vi "Write Sync Group.vi"(8 "error in (no error)":errorcluster, 10 "Sync Group":u8=128 format="%x", 11 "DriveMotorsLeft in":refnum<class "DriveMotorsLeft.lvclass">) -> (0 "error out":errorcluster, 3 "DriveMotorsLeft out":refnum<class "DriveMotorsLeft.lvclass">)   [LabVIEW 2013, in "DriveMotorsLeft.lvclass"]
uses:
  DriveMotorsLeft.lvclass
  DriveMotorsLeft.lvclass/DriveMotorsLeft.ctl
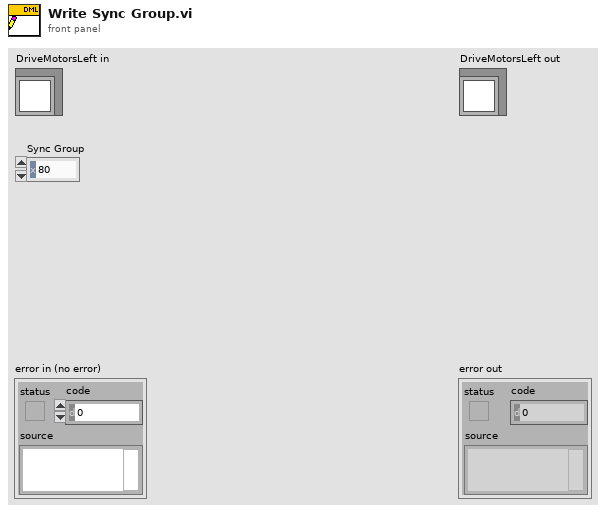
[diagram p1: front panel]
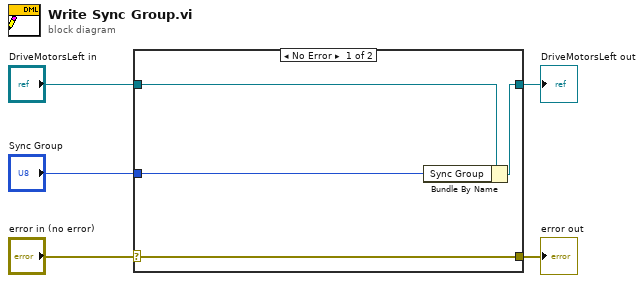
[diagram p0: block diagram]
diagram:
  n1 = case shown="No Error" "error in (no error)" {
    selector: "error in (no error)" -> [w9 w10]
    tunnel: [w9 w10] -> w4
    tunnel: [w7 w11] -> w2
    tunnel: "DriveMotorsLeft in" -> [w8 w11]
    tunnel: "Sync Group" -> [w6 _]
    frame No Error {
      n2 = Bundle By Name(cluster=w8, "Sync Group"=w6) -> (w7:refnum<class "DriveMotorsLeft.lvclass">)
    }
    frame Error {
    }
  }
  "error out" <- w4
  "DriveMotorsLeft out" <- w2
